vi "TCP Server Engine.vi"(8 "error in (no error)":errorcluster, 9 "User Events":T1, 10 "Port (0)":i32, 11 "Service Name":string) -> (0 "error out":errorcluster)   [LabVIEW 2016, in "SLL Easy API via TCP.lvclass"]
uses:
  SLL Easy API via TCP.lvclass
  _Typedefs/User Events to TCP Engine.ctl
  _Typedefs/TCP Event Data.ctl
  <vilib>/Utility/error.llb/DialogType.ctl
  SLL Queued State Machine/Queue Driver/Create Queue.vi
  SLL Queued State Machine/Queue Driver/Enqueue an Item to Queue.vi
  SLL Queued State Machine/Queue Driver/Dequeue Queue.vi
  SLL Queued State Machine/Queue Driver/Enqueue N Items.vi
  SLL Queued State Machine/Queue Driver/Flush Queue.vi
  SLL Queued State Machine/Queue Driver/Release Queue.vi
  SLL Queued State Machine/SLL QSM.lvlib
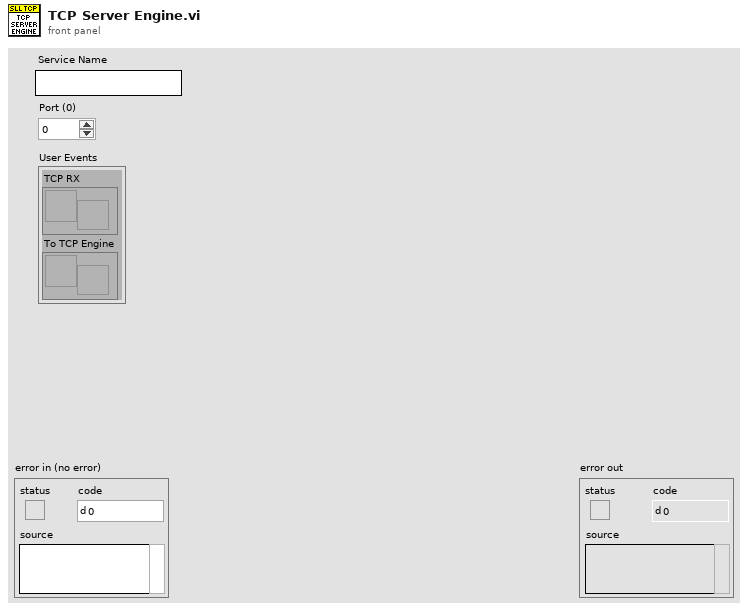
[diagram p1: front panel]
types:
  T1 = typedef "SLL Easy API via TCP.lvclass/User Events to TCP Engine.ctl" = cluster{"TCP RX":refnum<user-event>, "To TCP Engine":refnum<user-event>}
  T2 = cluster{"Flags":cluster{"Source Code?":bool}, "Listener ID":refnum<k5>, "Connection ID[]":refnum<k5>[], "User Events":T1}
  T3 = typedef "DialogType.ctl" = u16
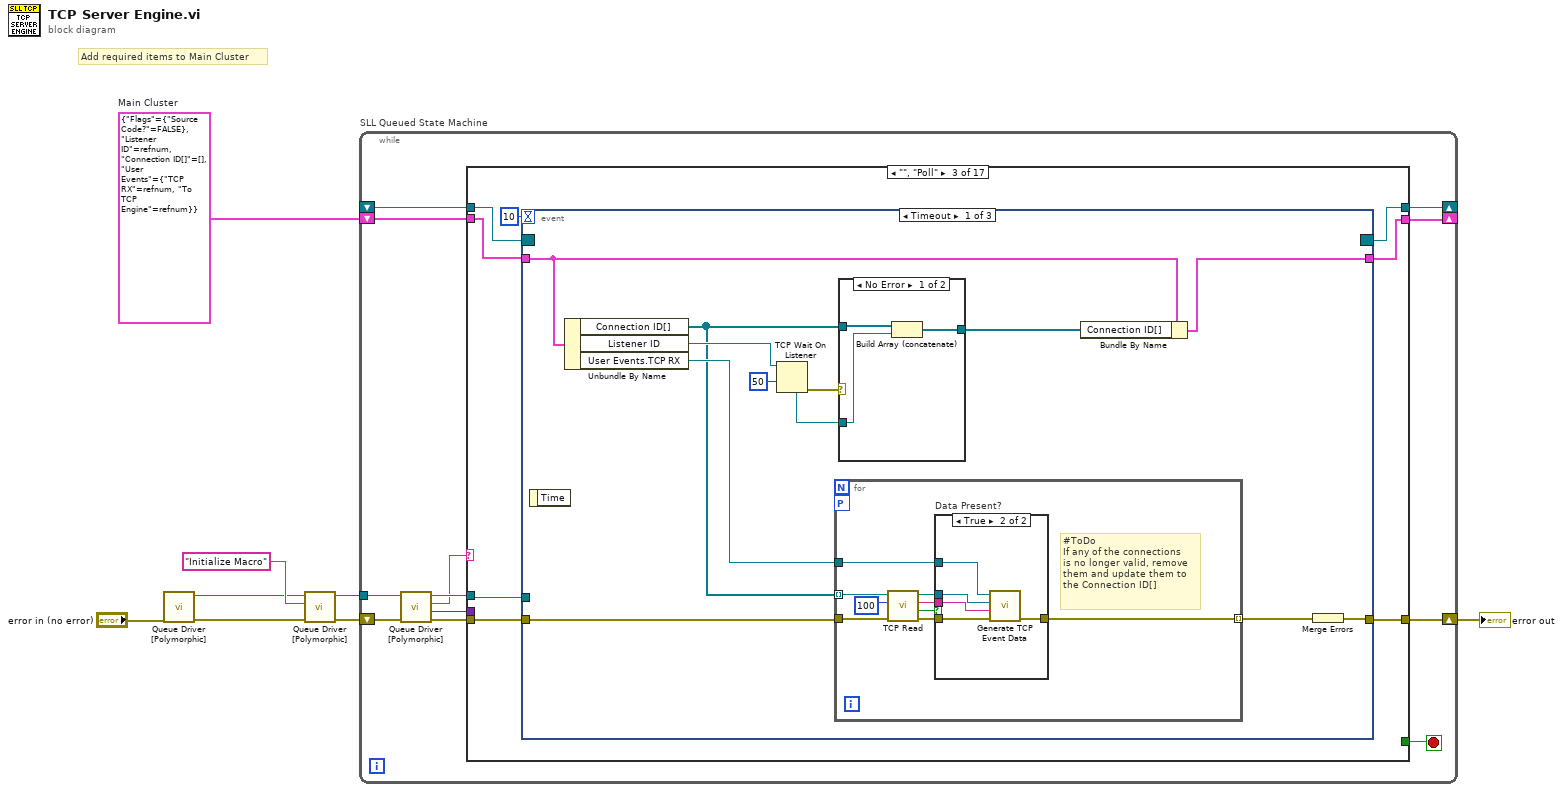
[diagram p0: block diagram]
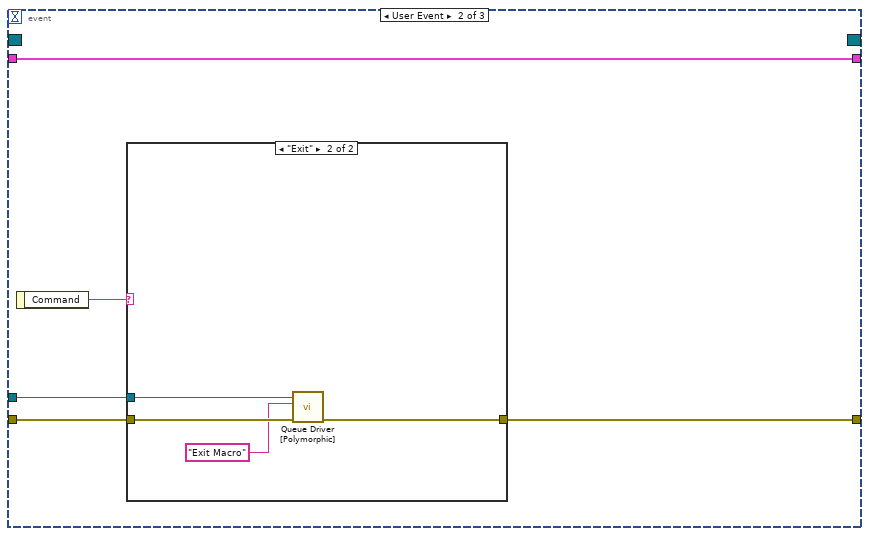
[diagram p6: hidden frame]
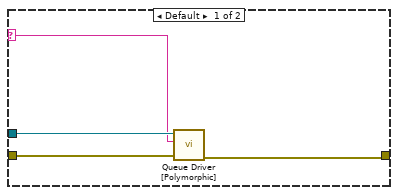
[diagram p7: hidden frame]
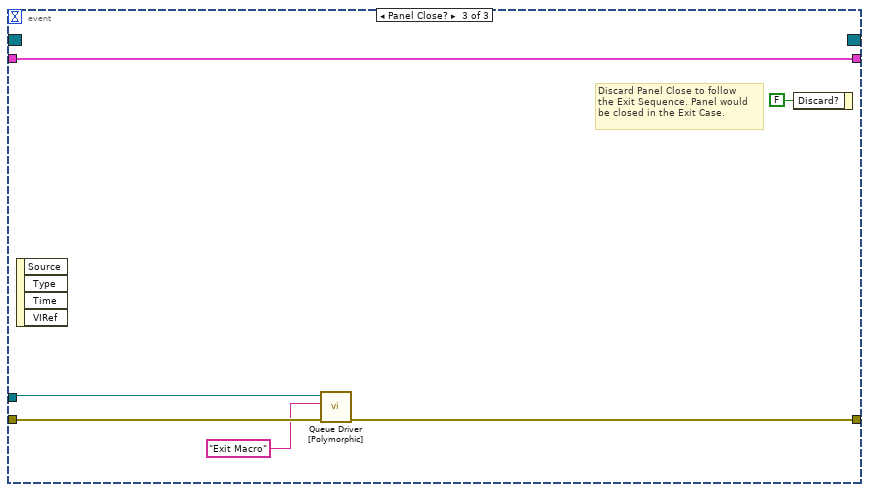
[diagram p8: hidden frame]
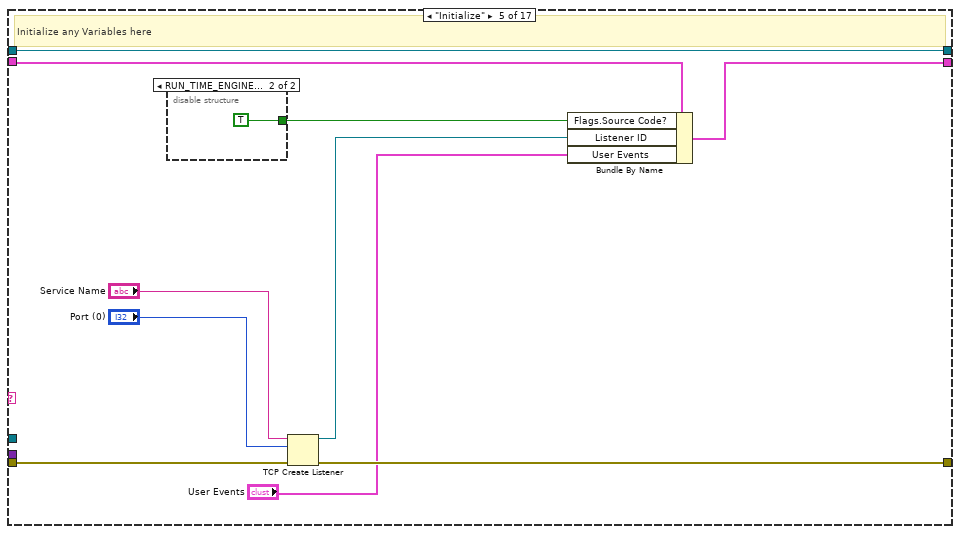
[diagram p10: hidden frame]
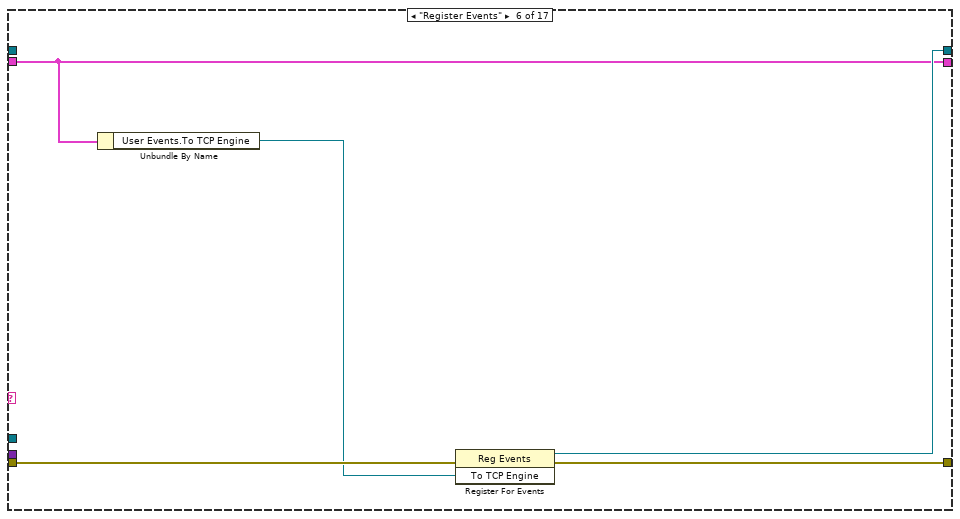
[diagram p12: hidden frame]
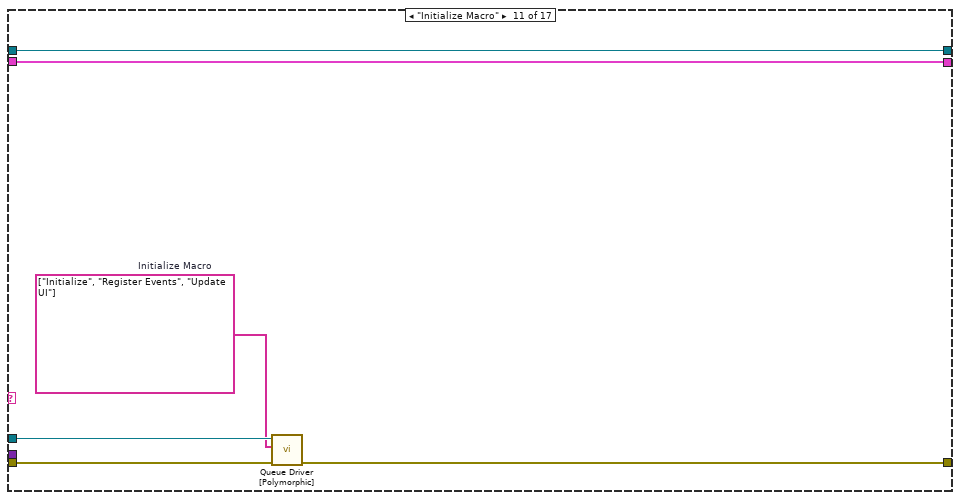
[diagram p17: hidden frame]
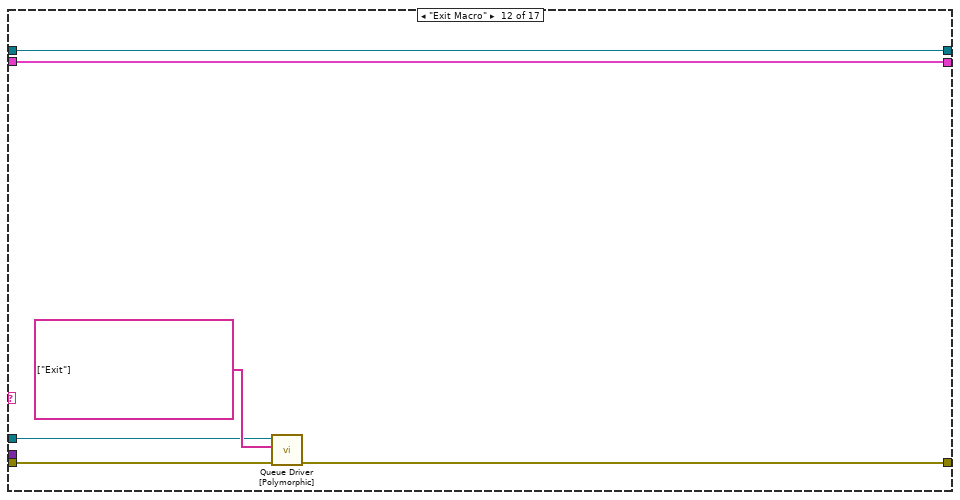
[diagram p18: hidden frame]
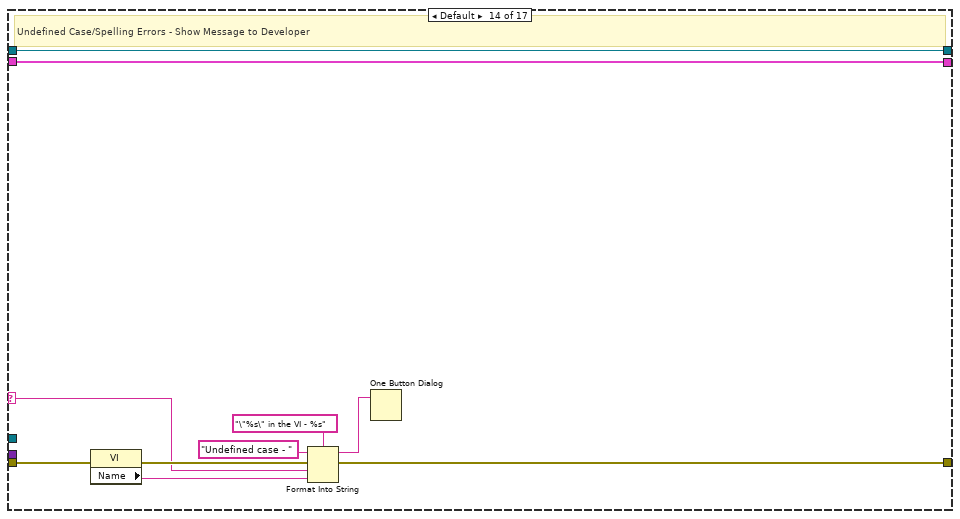
[diagram p20: hidden frame]
diagram:
  w8 = T2 {"Flags"={"Source Code?"=FALSE}, "Listener ID"=refnum, "Connection ID[]"=[], "User Events"={"TCP RX"=refnum, "To TCP Engine"=refnum}}  # Main Cluster
  # "Add required items to Main Cluster"
  n1 = call-poly "Queue Driver [Polymorphic].vi"("Error In"="error in (no error)") -> ("Error Out"=w6:errorcluster, "Queue Ref"=w2:refnum<queue>)  [unwired: 9 in]
  n2 = call-poly "Queue Driver [Polymorphic].vi"("Error In"=w6, "Item to Add"="Initialize Macro", "Queue Ref In"=w2) -> ("Error Out"=w7:errorcluster, "Queue Ref Out"=w1:refnum<queue>)  [unwired: 7 in]
  n3 = while "SLL Queued State Machine" {
    shift-right: [w18] -> w4
    shift-left: w7 -> [w20]
    shift-right: [w15] -> _
    shift-left: _ -> [w14]
    shift-right: [w13] -> _
    shift-left: w8 -> [w12]
    tunnel: w1 -> [w10]
    stop <- w17 stop-if-true
    n4 = call-poly "Queue Driver [Polymorphic].vi"("Error In"=w20, "Queue Ref In"=w10) -> ("Error Out"=w19:errorcluster, "Data"=w9:variant, "Dequeue"=w11:string, "Queue Ref Out"=w16:refnum<queue>)  [unwired: 6 in]
    n5 = case "QSM Case Structure" shown="\"\", \"Poll\"" w11 {
      selector: w11 -> [_ _ _ _ _ _ _ _ _ _ _ _ _ w131 _ _ _]
      tunnel: w19 -> [w23 w26 w32 w87 w93 w103 w106 w109 w112 w115 w119 w125 w130 w134 w146 w149 w162]
      tunnel: [w23 w26 w33 w87 w92 w102 w106 w109 w112 w115 w118 w124 w130 w137 w144 w149 w158] -> w18
      tunnel: [_ _ _ _ _ _ _ _ _ _ _ _ _ _ _ _ TRUE] -> w17
      tunnel: [w22 w25 w31 w86 w97 w101 w105 w108 w111 w114 w121 w127 w129 w140 w143 w148 w161] -> w15
      tunnel: w14 -> [w22 w25 w30 w86 w97 _ w105 w108 w111 w114 w121 w127 w129 w140 w143 w148 w161]
      tunnel: [w21 w24 w28 w85 w94 w100 w104 w107 w110 w113 w120 w126 w128 w139 w142 w147 w160] -> w13
      tunnel: w12 -> [w21 w24 w29 w85 w95 w100 w104 w107 w110 w113 w120 w126 w128 w139 w142 w147 w160]
      tunnel: w16 -> [_ _ w27 _ _ _ _ _ _ _ w117 w122 _ _ _ _ w151]
      tunnel: w9 -> [_ _ _ _ _ _ _ _ _ _ _ _ _ _ _ _ _]
      frame "/*** Read Me ***/" {
        # "General Purpose Queue Based State Machine for Any Use Case (main application, module, pop up message etc)\n\nAdvantages:\n1. No Need to Pass Queue References between Queue Driver VIs.\n2. This template can be safely used in multiple parallel running modules without any issues.\n3. This template can also be safely used even in cases where the VI is configured to be a Clone, where multiple \ninstances of the VI could be executing concurrently.\n\nHow to Use:\n1. Add necessary items to the Main Cluster.\n2. Use the Polymorphic Queue Driver for doing any queue operations. There is no need to pass the queue driver\nreference, as the Queue Driver automatically infers the reference based on the VI instance from which it is called.\n3. Add any required user events in the \"Register Events\" case. Ignore if not needed.\n4. Use \"Sequences\" section for defining any list of state calls, which could be used in multiple places. \nEg: Initialize Sequence, might be needed if we need to any reinitialization."
      }
      frame "/**** Poll ****/" {
      }
      frame "", "Poll" {
        n6 = event shown="[0] Timeout" {
          selector: w30 -> [_ _ _]
          dyn-events: [_ _ _] -> w31
          timeout: 10 -> [_ _ _]
          tunnel: [w37 w68 w83] -> w33
          tunnel: w32 -> [w39 w69 w84]
          tunnel: w29 -> [w42 w70 w82]
          tunnel: [w41 w70 w82] -> w28
          tunnel: w27 -> [_ w66 w80]
          event Timeout {
            n7 = event-data() -> ()  [unwired: 1 in, 1 out]
            n8 = Unbundle By Name(w42) -> ("Connection ID[]"=w35:refnum<k5>[], "Listener ID"=w46:refnum<k5>, "User Events.TCP RX"=w36:refnum<user-event>)
            n9 = TCP Wait On Listener(9:50 ("timeout ms (wait forever: -1)"), 11:w46) -> (0:w44:errorcluster, 4:w43:refnum<k5>)  [unwired: 2 in, 3 out]
            n10 = for {
              tunnel: w35 -> [w55] mode=indexing
              workers-P: _ -> [_]
              tunnel: w39 -> [w54]
              tunnel: [w52] -> w38 mode=indexing
              tunnel: w36 -> [w48]
              # "#ToDo\nIf any of the connections\nis no longer valid, remove\nthem and update them to\nthe Connection ID[]"
              n11 = call "TCP Read.vi"("error in (no error)"=w54, "timeout ms (1000)"=100, "Connection ID In"=w55) -> ("error out"=w53:errorcluster, "Data Available?"=w50:bool, "Read Data"=w51:string, "Connection ID Out"=w49:refnum<k5>)  [unwired: 5 in]
              n12 = case "Data Present?" shown="True" w50 {
                tunnel: w53 -> [w56 w61]
                tunnel: [w56 w60] -> w52
                tunnel: w51 -> [_ w57]
                tunnel: w48 -> [_ w59]
                tunnel: w49 -> [_ w58]
                frame False {
                }
                frame True {
                  n13 = call "Generate TCP Event Data.vi"("error in (no error)"=w61, "TCP Data"=w57, "Connection ID"=w58, "User Events.TCP RX"=w59) -> ("error out"=w60:errorcluster)  [unwired: 7 in]
                }
              }
            }
            n14 = case shown="No Error" w44 {
              tunnel: w35 -> [w64 w65]
              tunnel: w43 -> [w63 _]
              tunnel: [w62 w65] -> w40
              frame No Error {
                n15 = Build Array (concatenate)(w64, w63) -> (w62:refnum<k5>[])
              }
              frame Error {
              }
            }
            n16 = Bundle By Name(cluster=w42, "Connection ID[]"=w40) -> (w41:T2)
            n17 = Merge Errors(w38) -> (w37:errorcluster)
          }
          event User Event {
            n18 = event-data() -> ("Command"=w67:string)  [unwired: 1 in]
            n19 = case shown="\"Exit\"" w67 {
              selector: w67 -> [w71 _]
              tunnel: w69 -> [w74 w78]
              tunnel: [w73 w77] -> w68
              tunnel: w66 -> [w72 w76]
              frame Default {
                n20 = call-poly "Queue Driver [Polymorphic].vi"("Error In"=w74, "Item to Add"=w71, "Queue Ref In"=w72) -> ("Error Out"=w73:errorcluster)  [unwired: 7 in, 1 out]
              }
              frame "Exit" {
                n21 = call-poly "Queue Driver [Polymorphic].vi"("Error In"=w78, "Item to Add"="Exit Macro", "Queue Ref In"=w76) -> ("Error Out"=w77:errorcluster)  [unwired: 7 in, 1 out]
              }
            }
          }
          event Panel Close? {
            # "Discard Panel Close to follow\nthe Exit Sequence. Panel would\nbe closed in the Exit Case."
            n22 = event-data() -> ()  [unwired: 1 in, 4 out]
            n23 = call-poly "Queue Driver [Polymorphic].vi"("Error In"=w84, "Item to Add"="Exit Macro" ("Enqueue"), "Queue Ref In"=w80) -> ("Error Out"=w83:errorcluster)  [unwired: 7 in, 1 out]
            n24 = event-data("Discard?"=FALSE) -> ()  [unwired: 1 in, 1 out]
          }
        }
      }
      frame "/**** Initialize ****/" {
      }
      frame "Initialize" {
        # "Initialize any Variables here"
        n25 = disable-structure shown="RUN_TIME_ENGINE==False" {
          disable-tunnel: [_ TRUE] -> w96
          frame condition #0 {
          }
          frame condition #1 (active) {
          }
        }
        n26 = TCP Create Listener(8:w93, 10:"Port (0)", 11:"Service Name") -> (0:w92:errorcluster, 3:w89:refnum<k5>)  [unwired: 2 in, 1 out]
        n27 = Bundle By Name(cluster=w95, "Flags.Source Code?"=w96, "Listener ID"=w89, "User Events"="User Events") -> (w94:T2)
      }
      frame "Register Events" {
        n28 = Unbundle By Name(w100) -> ("User Events.To TCP Engine"=w99:refnum<user-event>)
        n29 = register-events(error in=w103, w99) -> (reference out=w101:refnum<event-registration>, error out=w102:errorcluster)  [unwired: 1 in]
      }
      frame "/*** Custom Case Splitter ***/" {
      }
      frame "/*** User Interface Actions ***/" {
        # "Duplicate this case to create additional case splitters for readability"
      }
      frame "Update UI" {
        # "Update Front Panel Controls in this Case"
      }
      frame "/*** Macros ***/" {
      }
      frame "Initialize Macro" {
        w116 = string[] ["Initialize", "Register Events", "Update UI"]  # Initialize Macro
        n30 = call-poly "Queue Driver [Polymorphic].vi"("Error In"=w119, "Enqueue N"=w116, "Queue Ref In"=w117) -> ("Error Out"=w118:errorcluster)  [unwired: 7 in, 1 out]
      }
      frame "Exit Macro" {
        n31 = call-poly "Queue Driver [Polymorphic].vi"("Error In"=w125, "Enqueue N"=string[] ["Exit"], "Queue Ref In"=w122) -> ("Error Out"=w124:errorcluster)  [unwired: 7 in, 1 out]
      }
      frame "/*** Error Handler ***/" {
      }
      frame Default {
        # "Undefined Case/Spelling Errors - Show Message to Developer"
        n32 = property class="VI"(error in=w134) -> (error out=w133:errorcluster, "Name"=w132:string)  [unwired: 1 in, 1 out]
        n33 = Format Into String(format string="\"%s\" in the VI - %s" ("message"), initial string="Undefined case - ", error in=w133, w131, w132) -> (resulting string=w135:string, error out=w137:errorcluster)
        n34 = One Button Dialog(message=w135) -> ()  [unwired: 1 in, 1 out]
      }
      frame "Error" {
        w141 = T3 2 items=["no dialog", "OK message", "continue or stop message", "OK message + warnings", "continue/stop + warnings"] ("type of dialog (OK msg:1)")
        # "Handle the Error"
        n35 = call <vilib>:"Simple Error Handler.vi"("type of dialog (OK msg:1)"=w141, "error in (no error)"=w146) -> ("error out"=w145:errorcluster)  [unwired: 3 in, 4 out]
        n36 = call <vilib>:"Clear Errors.vi"("error in (no error)"=w145) -> ("error out"=w144:errorcluster)  [unwired: 5 in, 1 out]
      }
      frame "/**** Exit ****/" {
      }
      frame "Exit" {
        n37 = call-poly "Queue Driver [Polymorphic].vi"("Error In"=w162, "Queue Ref In"=w151) -> ("Error Out"=w163:errorcluster, "Queue Ref Out"=w150:refnum<queue>)  [unwired: 7 in, 1 out]
        n38 = Unbundle By Name(w160) -> ("Flags.Source Code?"=w153:bool)
        n39 = call-poly "Queue Driver [Polymorphic].vi"("Error In"=w163, "Queue Ref In"=w150) -> ("Error Out"=w159:errorcluster)  [unwired: 9 in]
        n40 = Call Chain() -> (call chain=w157:string[])
        n41 = Array Size(array=w157) -> (size(s)=w156:i32)
        n42 = Equal?(x=w156, y=1) -> (x = y?=w154:bool)
        n43 = And(x=w153, y=w154) -> (x .and. y?=w152:bool)
        n44 = case "Skip Panel Close when in Source\nCode and is the top most caller" shown="True" w152 {
          tunnel: w159 -> [w166 w168]
          tunnel: [w167 w168] -> w158
          frame False {
            # "Close Panel"
            n45 = invoke class="VI" method="FP.Close"() -> (error out=w165:errorcluster)  [unwired: 3 in, 2 out]
            n46 = Merge Errors(w166, w165) -> (w167:errorcluster)
          }
          frame True {
            # "Do Not Close Panel"
          }
        }
      }
    }
  }
  "error out" <- w4
